vi "Untitled 3.vi"() -> ()   [LabVIEW 2014]
panel:
  out "Força":dbl(knob) scale=0.0..50.0
  in  "Ciclo 2":dbl(slide) scale=0.0..10.0
  out "Vibração":cluster{"X":dbl, "Y":dbl}[](graph)
  in  "Ciclo 1":dbl(slide) scale=0.0..10.0
  out "Rotação":dbl(knob) scale=0.0..800.0
  out "Termopar Ref":dbl[unit](slide)=273.15 scale=273.15..333.15
  out "Termopar B":dbl[unit](slide)=273.15 scale=273.15..873.15
  out "Termopar A":dbl[unit](slide)=273.15 scale=273.15..873.15
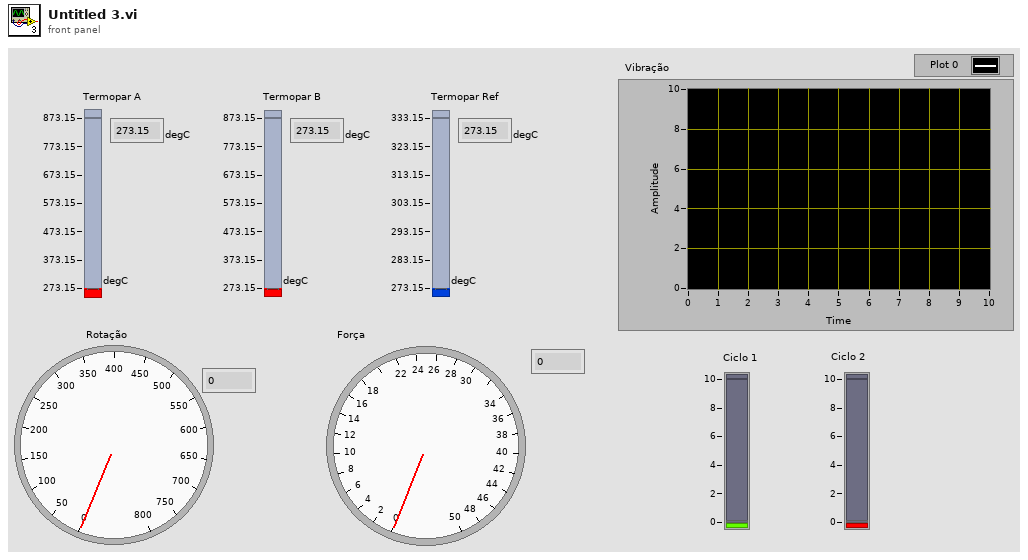
[diagram p1: front panel]
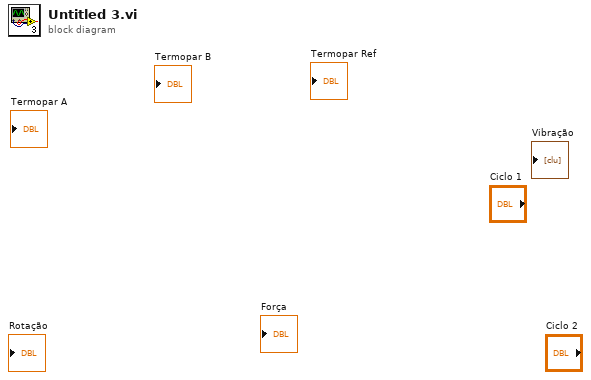
[diagram p0: block diagram]
diagram:
